vi "Read Initialized.vi"(8 "error in (no error)":errorcluster, 11 "Device Data Model in":refnum<class "Device Data Model.lvclass">) -> (0 "error out":errorcluster, 2 "Initialized":bool, 3 "Device Data Model out":refnum<class "Device Data Model.lvclass">)   [LabVIEW 2012, in "Device Data Model.lvclass"]
uses:
  Device Data Model.lvclass
  Device Data Model.lvclass/Device Data Model.ctl
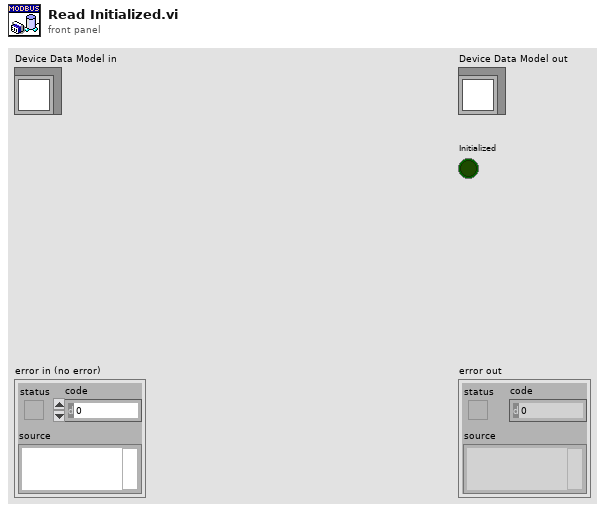
[diagram p1: front panel]
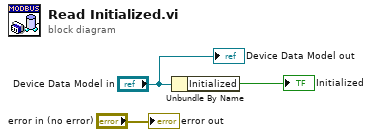
[diagram p0: block diagram]
diagram:
  n1 = Unbundle By Name("Device Data Model in") -> ("Initialized"=→"Initialized":bool)
  "error out" <- "error in (no error)"
  "Device Data Model out" <- "Device Data Model in"
